vi "Write Command.vi"(8 "error in (no error)":errorcluster, 10 "Command":string, 11 "Sync Box in":refnum<class "Sync Box.lvclass">) -> (0 "error out":errorcluster, 3 "Sync Box out":refnum<class "Sync Box.lvclass">)   [LabVIEW 2018, in "Sync Box.lvclass"]
uses:
  Sync Box.lvclass
  Sync Box.lvclass/Sync Box.ctl
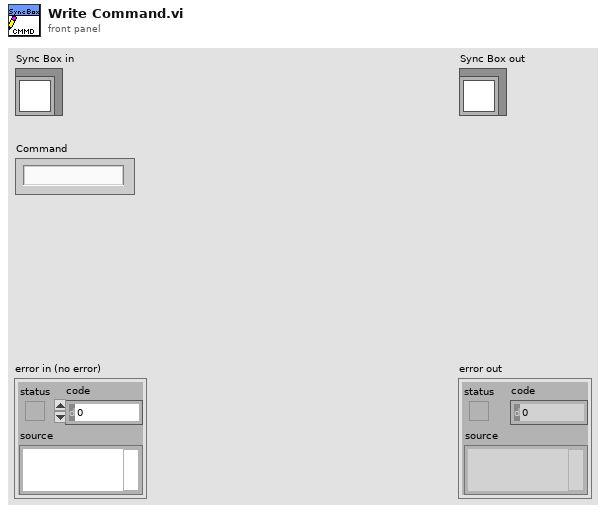
[diagram p1: front panel]
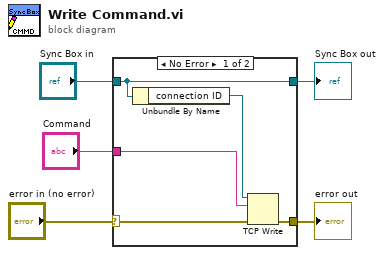
[diagram p0: block diagram]
diagram:
  n1 = case shown="No Error" "error in (no error)" {
    selector: "error in (no error)" -> [w9 w11]
    tunnel: [w10 w11] -> w4
    tunnel: [w8 w12] -> w2
    tunnel: "Sync Box in" -> [w8 w12]
    tunnel: "Command" -> [w6 _]
    frame No Error {
      n2 = Unbundle By Name(w8) -> ("connection ID"=w7:refnum<k5>)
      n3 = TCP Write(connection ID=w7, data in=w6, error in (no error)=w9) -> (error out=w10:errorcluster)  [unwired: 1 in, 2 out]
    }
    frame Error {
    }
  }
  "error out" <- w4
  "Sync Box out" <- w2
